vi "Check Equipment.vi"(8 "error in (no error)":errorcluster, 10 "Bit Mask":u32 format="%.0x", 11 "VISA resource name":refnum<visa-resource-name>) -> (0 "error out":errorcluster {"code" format="%.0x"}, 2 "Present?":u32, 3 "VISA resource name out":refnum<visa-resource-name>)   [LabVIEW 2012, in "Fluke 5XXX Series Multicalibrators.lvlib"]
doc: "This VI returns the instrument specific attributes (instrument model, instrument option and check status) to a value corresponding to the present instrument."
uses:
  Fluke 5XXX Series Multicalibrators.lvlib
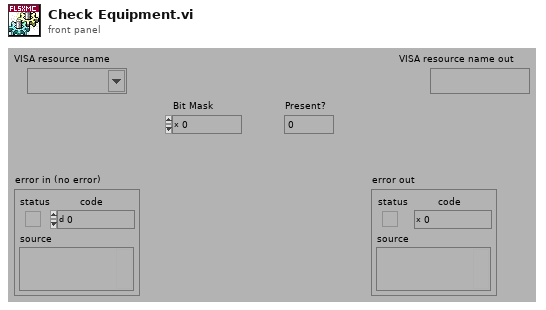
[diagram p1: front panel]
types:
  T1 = cluster{"Status":bool, "Code":i32, "Source (VI Name)":string}
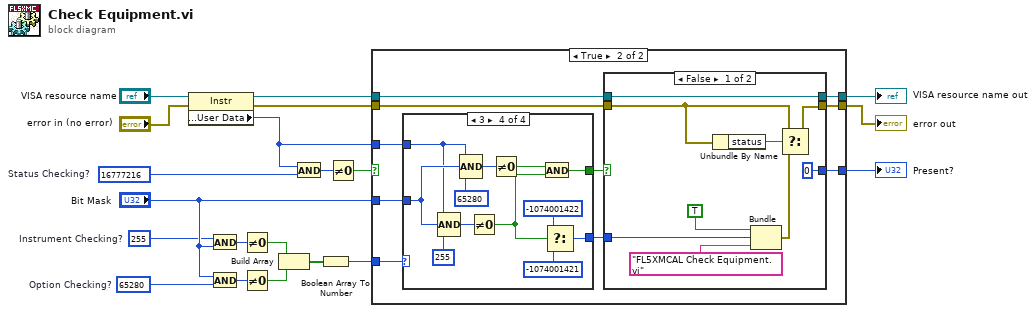
[diagram p0: block diagram]
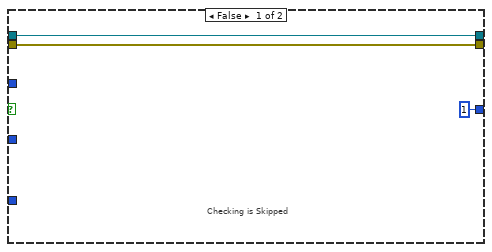
[diagram p2: hidden frame]
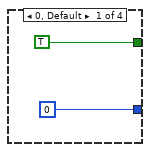
[diagram p3: hidden frame]
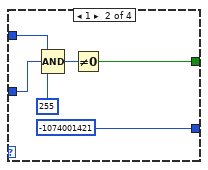
[diagram p4: hidden frame]
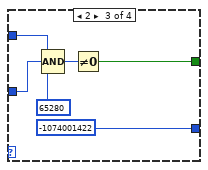
[diagram p5: hidden frame]
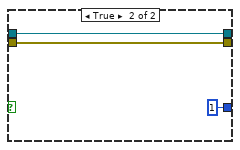
[diagram p6: hidden frame]
diagram:
  w15 = u32 65280  # Option Checking?
  w6 = u32 255  # Instrument Checking?
  w18 = u32 16777216  # Status Checking?
  n1 = property class="Instr"(reference="VISA resource name", error in="error in (no error)") -> (reference out=w4:refnum<visa-resource-name>, error out=w2:errorcluster, "General Settings:User Data"=w1:u32)
  n2 = And(x=w6, y="Bit Mask") -> (x .and. y?=w8:u32)
  n3 = And(x="Bit Mask", y=w15) -> (x .and. y?=w9:u32)
  n4 = Not Equal To 0?(x=w8) -> (x != 0?=w13:bool)
  n5 = Not Equal To 0?(x=w9) -> (x != 0?=w11:bool)
  n6 = Build Array(w13, w11) -> (w14:bool[])
  n7 = And(x=w1, y=w18) -> (x .and. y?=w16:u32)
  n8 = Boolean Array To Number(Boolean array=w14) -> (number=w12:u32)
  n9 = Not Equal To 0?(x=w16) -> (x != 0?=w10:bool)
  n10 = case shown="True" w10 {
    tunnel: [u32 1 w29] -> w20
    tunnel: w1 -> [_ w27]
    tunnel: w2 -> [w22 w33]
    tunnel: [w23 w30] -> w19
    tunnel: w4 -> [w23 w31]
    tunnel: [w22 w32] -> w17
    tunnel: w12 -> [_ w28]
    tunnel: "Bit Mask" -> [_ w24]
    frame False {
      # "Checking is Skipped"
    }
    frame True {
      n11 = case shown="3" w28 {
        tunnel: w27 -> [_ w40 w46 w55]
        tunnel: [TRUE w38 w44 w53] -> w26
        tunnel: [0 ("Code") -1074001421 ("Code") -1074001422 ("Code") w51] -> w25
        tunnel: w24 -> [_ w37 w43 w56]
        frame 0, Default {
        }
        frame 1 {
          n12 = Compound Arithmetic op=AND(w40, w37, u32 255 ("Instrument Checking?")) -> (w39:u32)
          n13 = Not Equal To 0?(x=w39) -> (x != 0?=w38:bool)
        }
        frame 2 {
          n14 = Compound Arithmetic op=AND(w46, w43, u32 65280 ("Option Checking?")) -> (w45:u32)
          n15 = Not Equal To 0?(x=w45) -> (x != 0?=w44:bool)
        }
        frame 3 {
          n16 = Compound Arithmetic op=AND(w55, w56, u32 255 ("Instrument Checking?")) -> (w57:u32)
          n17 = Compound Arithmetic op=AND(w55, w56, u32 65280 ("Option Checking?")) -> (w59:u32)
          n18 = Not Equal To 0?(x=w57) -> (x != 0?=w48:bool)
          n19 = Not Equal To 0?(x=w59) -> (x != 0?=w52:bool)
          n20 = And(x=w52, y=w48) -> (x .and. y?=w53:bool)
          n21 = Select(t=-1074001422 ("Code"), s=w48, f=-1074001421 ("Code")) -> (s? t:f=w51:i32)
        }
      }
      n22 = case shown="False" w26 {
        tunnel: w33 -> [w65 w71]
        tunnel: [w63 w71] -> w32
        tunnel: [w64 w70] -> w30
        tunnel: w31 -> [w64 w70]
        tunnel: [u32 0 u32 1] -> w29
        tunnel: w25 -> [w60 _]
        frame False {
          n23 = Unbundle By Name(w65) -> ("status"=w61:bool)
          n24 = Bundle("Status"=TRUE, "Code"=w60, "Source (VI Name)"="FL5XMCAL Check Equipment.vi") -> (w67:T1)  [unwired: 1 in]
          n25 = Select(t=w65, s=w61, f=w67) -> (s? t:f=w63:T1)
        }
        frame True {
        }
      }
    }
  }
  "error out" <- w17
  "VISA resource name out" <- w19
  "Present?" <- w20
